vi "00 - Built-in Processing.vi"() -> ()   [LabVIEW 2021]
uses:
  <vilib>/Waveform/DWDTOps.llb/DWDT Search for Digital Pattern.vi
  <vilib>/Analysis/NI_AALPro.lvlib
  <vilib>/Analysis/7linalg.llb/Solve Linear Equations (single right hand).vi
  <vilib>/gmath/NI_Gmath.lvlib
  <vilib>/gmath/interp.llb/Interpolate 2D (2d X,Y).vi
  <vilib>/gmath/statdist.llb/Rayleigh Random.vi
  <vilib>/Analysis/NI_AALBase.lvlib
  <vilib>/Analysis/polynomials.llb/Polynomial Roots (DBL).vi
  <vilib>/Analysis/coordinate.llb/3D Cartesian Coordinate Rotation (Euler) (Array).vi
  <vilib>/Analysis/baseanly.llb/Matrix Type of Inverse Matrix.ctl
  <vilib>/Analysis/Matrix/Datatypes/RealMatrix.ctl
  <vilib>/Analysis/Matrix/NI_Matrix.lvlib
panel:
  out "transposed matrix":T1
  out "Solution Vector":dbl[](array[numeric]) format="%.2f"
  out "error":i32
  in  "Input Matrix":T1
  in  "Known Vector":dbl[](array[numeric]) format="%.2f"
  in  "matrix type":T2
  in  "integer":i32
  out "fixed-point":fxp<+,1,1> format="%.21g"
  out "r * e^(i*theta)":cdb[](array[numeric])
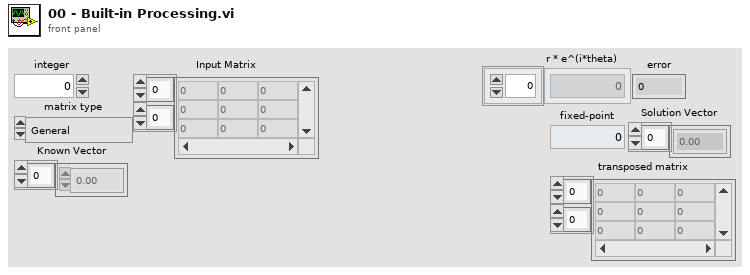
[diagram p1: front panel]
types:
  T1 = typedef "NI_Matrix.lvlib/RealMatrix.ctl" = dbl[][]
  T2 = typedef "NI_AALBase.lvlib/Matrix Type of Inverse Matrix.ctl" = enum32{"General", "Positive Definite", "Lower Triangular", "Upper Triangular"}
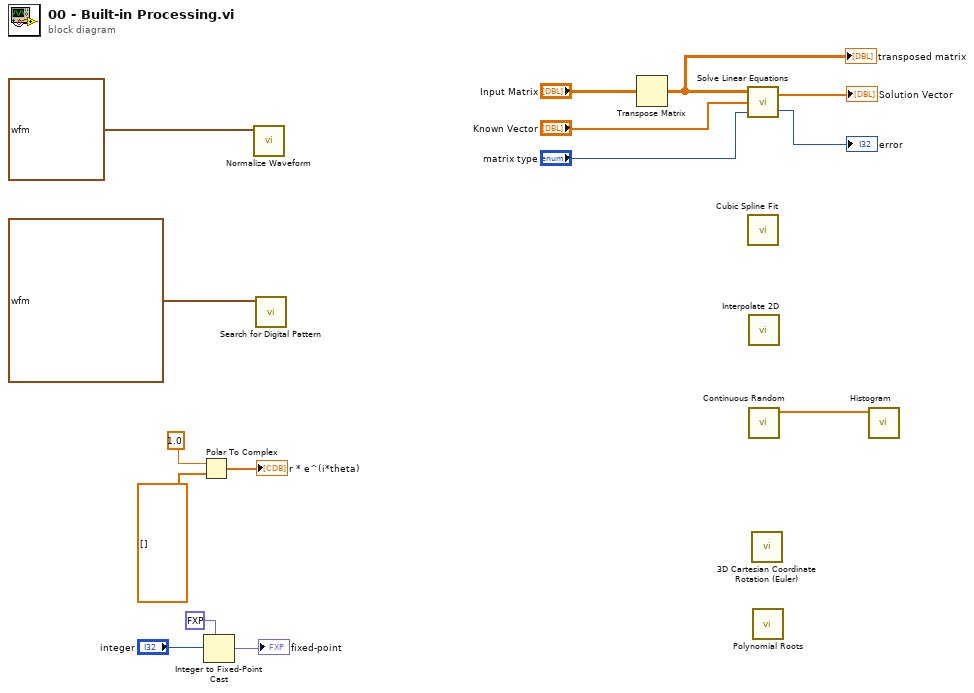
[diagram p0: block diagram]
diagram:
  n1 = Polar To Complex(1:dbl[] [] ("theta"), 2:1.0 ("r")) -> (0:→"r * e^(i*theta)":cdb[])
  n2 = Integer to Fixed-Point Cast(fixed-point type=fxp<+,1,1> 0.0, integer="integer") -> (fixed-point=→"fixed-point":fxp<+,1,1>)
  n3 = call <vilib>:"Normalize Waveform.vi"("waveform in"=waveform(dbl) {"t0"=timestamp(0 s since 1904-01-01), "dt"=1.0, "Y"=[]} ("Waveform")) -> ()  [unwired: 7 in, 4 out]
  n4 = call-poly <vilib>:"Search for Digital Pattern.vi"("digital waveform in"=digitalwaveform {"t0"=timestamp(0 s since 1904-01-01), "dt"=0.0, "Y"={"transitions"=[], "data"=[]}, "error"={"status"=FALSE, "code"=37421928, "source"=""}}) -> ()  [unwired: 8 in, 3 out]
  n5 = Transpose Matrix(1:"Input Matrix") -> (0:w2:T1)
  "transposed matrix" <- w2
  n6 = call-poly <vilib>:"Solve Linear Equations.vi"("matrix type"="matrix type", "Known Vector"="Known Vector", "Input Matrix"=w2) -> ("error"=→"error":i32, "Solution Vector"=→"Solution Vector":dbl[])
  n7 = call <vilib>:"Cubic Spline Fit.vi"() -> ()  [unwired: 14 in, 2 out]
  n8 = call-poly <vilib>:"Interpolate 2D.vi"() -> ()  [unwired: 8 in, 4 out]
  n9 = call-poly <vilib>:"Continuous Random.vi"() -> ("Rayleigh random data"=w1:dbl[])  [unwired: 10 in, 1 out]
  n10 = call-poly <vilib>:"3D Cartesian Coordinate Rotation (Euler).vi"() -> ()  [unwired: 8 in, 4 out]
  n11 = call-poly <vilib>:"Polynomial Roots.vi"() -> ()  [unwired: 10 in, 2 out]
  n12 = call <vilib>:"Histogram.vi"("X"=w1) -> ()  [unwired: 7 in, 4 out]
